vi "select signals.vi"(0 "Serial Port":refnum<visa-resource-name>, 9 "Signal 1":T1) -> (4 "Serial Port":refnum<visa-resource-name>, 10 "signals":enum16{"signal 1", "signals 1 and 2"}(ring), 14 "Signal 2":T1, 15 "Signal 1":T1)   [LabVIEW 2012]
uses:
  signal.ctl
panel:
  in  "Signal 2":T1
  in  "signals":enum16{"signal 1", "signals 1 and 2"}(ring)
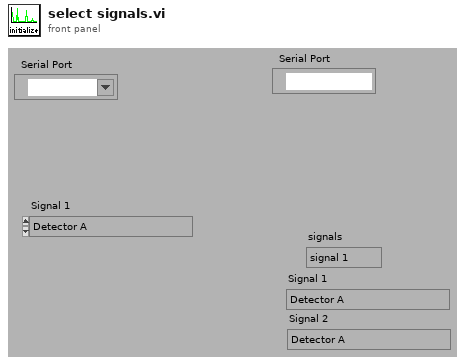
[diagram p1: front panel]
types:
  T1 = typedef "signal.ctl" = enum16{"Detector A", "Detector B", "Oven temperature", "Comp 1", "Comp 2", "Inlet A temperature", "Inlet B temperature", "Detector A temperature", "Detector B temperature", "Test Signal"}
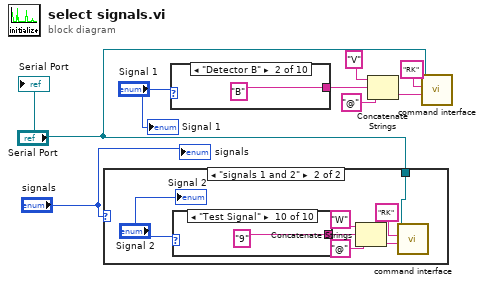
[diagram p0: block diagram]
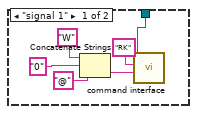
[diagram p2: hidden frame]
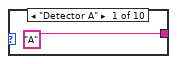
[diagram p3: hidden frame]
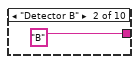
[diagram p4: hidden frame]
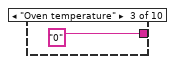
[diagram p5: hidden frame]
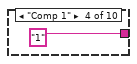
[diagram p6: hidden frame]
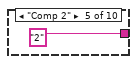
[diagram p7: hidden frame]
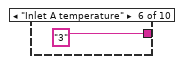
[diagram p8: hidden frame]
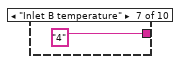
[diagram p9: hidden frame]
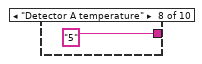
[diagram p10: hidden frame]
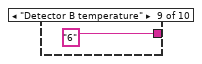
[diagram p11: hidden frame]
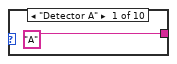
[diagram p12: hidden frame]
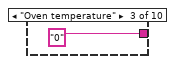
[diagram p13: hidden frame]
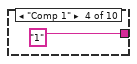
[diagram p14: hidden frame]
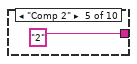
[diagram p15: hidden frame]
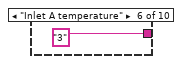
[diagram p16: hidden frame]
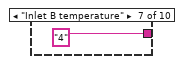
[diagram p17: hidden frame]
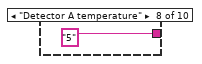
[diagram p18: hidden frame]
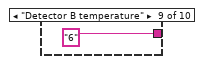
[diagram p19: hidden frame]
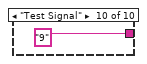
[diagram p20: hidden frame]
diagram:
  n1 = case shown="\"signals 1 and 2\"" "signals" {
    tunnel: "Serial Port" -> [w9 w21]
    frame "signal 1" {
      n2 = Concatenate Strings("W", "0", "@") -> (w14:string)
      n3 = call "command interface.vi"("Parameter"=w14, "command"="RK", "Serial Port"=w9) -> ()  [unwired: 4 in, 4 out]
    }
    frame "signals 1 and 2" {
      n4 = case shown="\"Test Signal\"" "Signal 2" {
        tunnel: ["A" "B" "0" "1" "2" "3" "4" "5" "6" "9"] -> w19
        frame "Detector A" {
        }
        frame "Detector B" {
        }
        frame "Oven temperature" {
        }
        frame "Comp 1" {
        }
        frame "Comp 2" {
        }
        frame "Inlet A temperature" {
        }
        frame "Inlet B temperature" {
        }
        frame "Detector A temperature" {
        }
        frame "Detector B temperature" {
        }
        frame "Test Signal" {
        }
      }
      n5 = Concatenate Strings("W", w19, "@") -> (w16:string)
      n6 = call "command interface.vi"("Parameter"=w16, "command"="RK", "Serial Port"=w21) -> ()  [unwired: 4 in, 4 out]
      "Signal 2" <- "Signal 2"
    }
  }
  n7 = case shown="\"Detector B\"" "Signal 1" {
    tunnel: ["A" "B" "0" "1" "2" "3" "4" "5" "6" "9"] -> w3
    frame "Detector A" {
    }
    frame "Detector B" {
    }
    frame "Oven temperature" {
    }
    frame "Comp 1" {
    }
    frame "Comp 2" {
    }
    frame "Inlet A temperature" {
    }
    frame "Inlet B temperature" {
    }
    frame "Detector A temperature" {
    }
    frame "Detector B temperature" {
    }
    frame "Test Signal" {
    }
  }
  n8 = Concatenate Strings("V", w3, "@") -> (w6:string)
  n9 = call "command interface.vi"("Parameter"=w6, "command"="RK", "Serial Port"="Serial Port") -> ()  [unwired: 4 in, 4 out]
  "Serial Port" <- "Serial Port"
  "signals" <- "signals"
  "Signal 1" <- "Signal 1"
